vi "Update Stats.vi"(8 "error in (no error)":errorcluster, 11 "SB App in":refnum<class "SB App.lvclass">) -> (0 "error out":errorcluster, 2 "Won?":bool, 3 "SB App out":refnum<class "SB App.lvclass">)   [LabVIEW 2020, in "SB App.lvlib" / "SB App.lvclass"]
uses:
  SB App.lvclass
  SB App.lvclass/SB App.ctl
  Dashboard Panel/Dashboard Panel.lvclass
  SquareBattle/Game/Game.lvclass
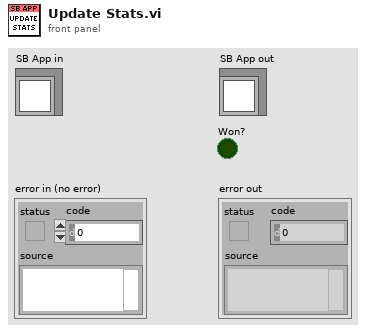
[diagram p1: front panel]
types:
  T1 = typedef "SB App.lvlib/Team Status Data.ctl" = cluster{"Team Stats":T2, "Team State":T3}
  T2 = typedef "SquareBattle.lvlib/Team Stats.ctl" = cluster{"Squares":i32, "Generated":i32, "Kills":i32, "Eliminated":i32, "Collisions":i32}
  T3 = typedef "SquareBattle.lvlib/Team State.ctl" = enum16{"Active", "Defeated", "Won"}
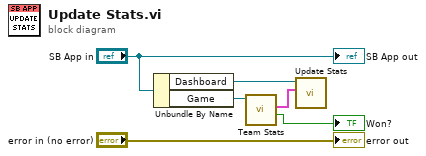
[diagram p0: block diagram]
diagram:
  n1 = Unbundle By Name("SB App in") -> ("Dashboard"=w4:refnum<class "Dashboard Panel.lvclass">, "Game"=w3:refnum<class "Game.lvclass">)
  n2 = call "Team Stats.vi"("Game in"=w3) -> ("Won?"=→"Won?":bool, "Team Stats"=w2:T1[])  [unwired: 7 in, 2 out]
  n3 = call "Update Stats.vi"("Team Stats"=w2, "Dashboard Panel in"=w4) -> ()  [unwired: 8 in, 2 out]
  "error out" <- "error in (no error)"
  "SB App out" <- "SB App in"
